vi "LogFileTimeDeb.vi"(4 "Input - Cluster":T2 {"Hysterese [°C]" format="%.2g"; "Dosiergeschw. [l/min]" format="%.2g"; "Dosiermenge [l]" format="%.2g"; "Druck I" format="%_3g"; "Füllstand  P" max=100 step=1 format="%#_3g"; "P-4 Drehzahl [%]" max=100 step=1 format="%#_3g"; "V-15 [%]" max=100 step=1 format="%_1g"; "V-13 [%]" max=100 step=1 format="%_1g"}, 5 "Actual Start [f] in":i64, 6 "Output - Cluster":T1 {"TS-5 [°C]" format="%#.2g"; "pHS-1 [pH]" format="%.2g"; "TS-4 [°C]" format="%#.2g"; "FS-2 [l]" format="%.2g"; "FS-1 [l]" format="%.2g"; "DS-1 [bar]" format="%#.2g"; "DFS-1 [l/min]" format="%#.2g"; "FS-3 [l]" format="%.2g"; "DFS-1 [dl]" format="%.0g"}, 7 "file Interval [s]":u32, 8 "error in (no error)":errorcluster, 9 "file":bool, 10 "file timing":i64, 11 "Byte Stream File in":refnum<file>) -> (0 "error out":errorcluster, 2 "Actual Start [f] out":i64, 3 "Byte Stream File out":refnum<file>)   [LabVIEW 2011]
uses:
  Input - Cluster b2g2.ctl
  Output - Cluster b2g2.ctl
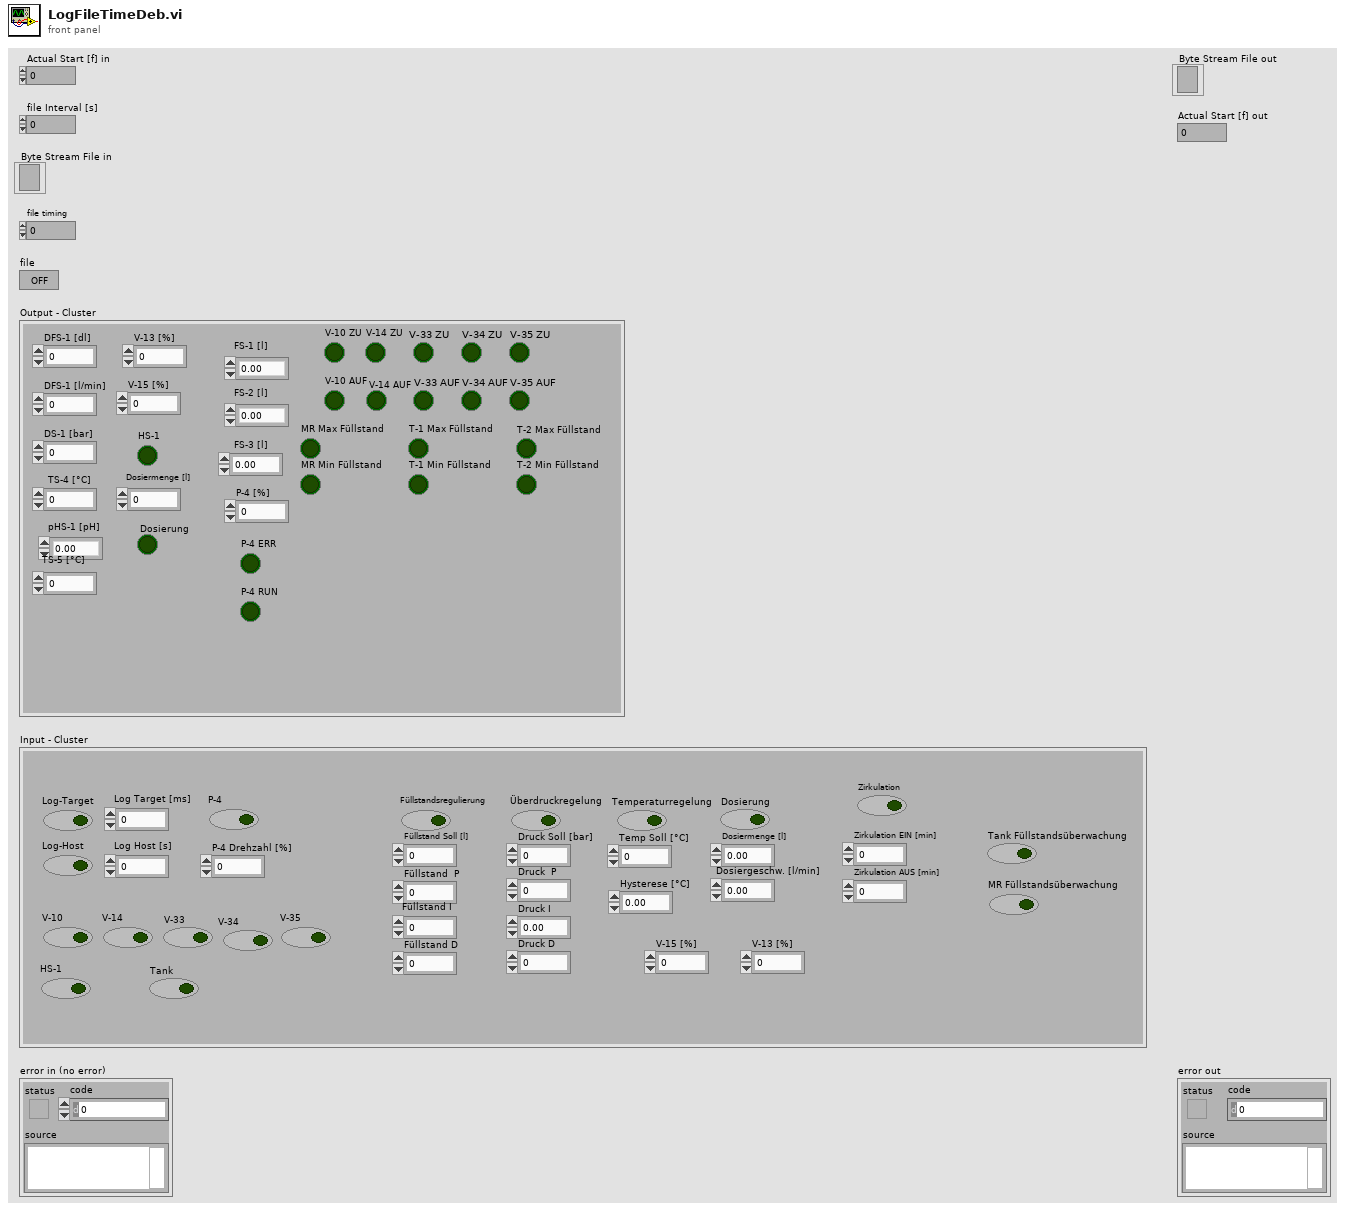
[diagram p1: front panel]
types:
  T1 = typedef "Output - Cluster b2g2.ctl" = cluster{"DFS-1 [dl]":u64, "FS-3 [l]":dbl, "DFS-1 [l/min]":dbl, "DS-1 [bar]":dbl, "V-10 ZU":bool, "V-14 ZU":bool, "FS-1 [l]":dbl, "FS-2 [l]":dbl, "TS-4 [°C]":dbl, "HS-1":bool, "V-13 [%]":u8, "V-15 [%]":u8, "P-4 [%]":u8, "Dosierung":bool, "MR Max Füllstand":bool, "MR Min Füllstand":bool, "Dosiermenge [l]":sgl, "V-14 AUF":bool, "V-10 AUF":bool, "T-1 Max Füllstand":bool, "T-1 Min Füllstand":bool, "T-2 Max Füllstand":bool, "T-2 Min Füllstand":bool, "pHS-1 [pH]":dbl, "P-4 RUN":bool, "V-33 AUF":bool, "V-33 ZU":bool, "V-34 AUF":bool, "V-34 ZU":bool, "P-4 ERR":bool, "TS-5 [°C]":dbl, "V-35 AUF":bool, "V-35 ZU":bool}
  T2 = typedef "Input - Cluster b2g2.ctl" = cluster{"V-13 [%]":u8, "V-15 [%]":u8, "Log-Target":bool, "P-4":bool, "P-4 Drehzahl [%]":u8, "Temperaturregelung":bool, "Überdruckregelung":bool, "Füllstandsregulierung":bool, "V-10":bool, "Log-Host":bool, "V-14":bool, "HS-1":bool, "Füllstand  P":sgl, "Füllstand I":sgl, "Füllstand D":sgl, "Füllstand Soll [l]":sgl, "Druck  P":sgl, "Druck I":sgl, "Druck D":sgl, "Druck Soll [bar]":sgl, "Temp Soll [°C]":sgl, "Dosierung":bool, "Dosiermenge [l]":sgl, "Dosiergeschw. [l/min]":sgl, "Tank":bool, "Hysterese [°C]":sgl, "MR Füllstandsüberwachung":bool, "Tank Füllstandsüberwachung":bool, "Log Target [ms]":u32, "Log Host [s]":u32, "Zirkulation EIN [min]":u8, "Zirkulation AUS [min]":u8, "Zirkulation":bool, "V-33":bool, "V-34":bool, "V-35":bool}
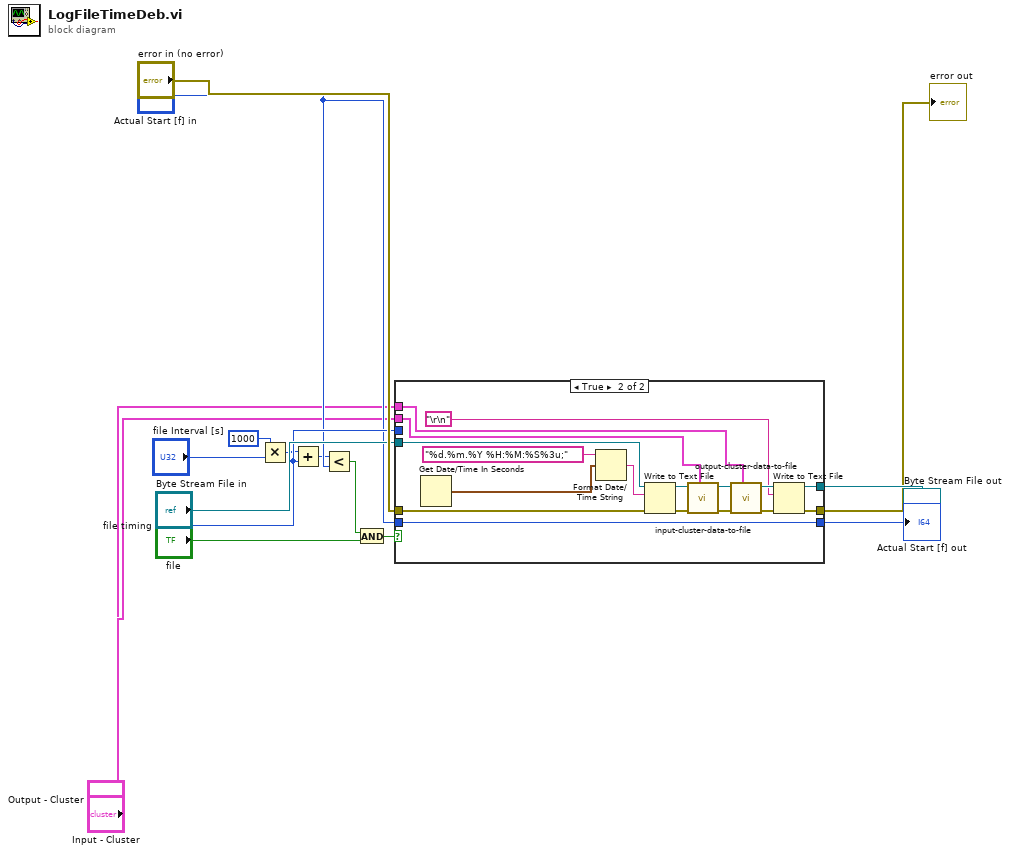
[diagram p0: block diagram]
diagram:
  n1 = Multiply(x=u32 1000, y="file Interval [s]") -> (x*y=w5:u32)
  n2 = Add(x=w5, y="file timing") -> (x+y=w2:i64)
  n3 = Less?(x=w2, y="Actual Start [f] in") -> (x < y?=w4:bool)
  n4 = And(x=w4, y="file") -> (x .and. y?=w3:bool)
  n5 = case shown="True" w3 {
    tunnel: [w17 w35] -> w15
    tunnel: [w18 w33] -> w14
    tunnel: [w19 w23] -> w16
    tunnel: "file timing" -> [w19 _]
    tunnel: "Output - Cluster" -> [_ w26]
    tunnel: "Input - Cluster" -> [_ w24]
    tunnel: "Actual Start [f] in" -> [_ w23]
    tunnel: "Byte Stream File in" -> [w17 w21]
    tunnel: "error in (no error)" -> [w18 w20]
    frame False {
    }
    frame True {
      n6 = Get Date/Time In Seconds() -> (seconds since 1Jan1904=w22:timestamp)
      n7 = Format Date/Time String(time format string (%c)="%d.%m.%Y %H:%M:%S%3u;", seconds (now)=w22) -> (date/time string=w27:string)  [unwired: 1 in]
      n8 = Write to Text File(file (use dialog)=w21, text=w27, error in=w20) -> (refnum out=w28:refnum<file>, error out=w29:errorcluster)  [unwired: 1 in, 1 out]
      n9 = call "input-cluster-data-to-file.vi"("refnum in"=w28, "error in"=w29, "Input - Cluster"=w24) -> ("refnum out"=w30:refnum<file>, "error out"=w25:errorcluster)  [unwired: 6 in]
      n10 = call "output-cluster-data-to-file.vi"("refnum in"=w30, "error in"=w25, "Output - Cluster"=w26) -> ("refnum out"=w36:refnum<file>, "error out"=w34:errorcluster)  [unwired: 6 in]
      n11 = Write to Text File(file (use dialog)=w36, text="\r\n", error in=w34) -> (refnum out=w35:refnum<file>, error out=w33:errorcluster)  [unwired: 1 in, 1 out]
    }
  }
  "Actual Start [f] out" <- w16
  "Byte Stream File out" <- w15
  "error out" <- w14
